vi "Save Data.vi"(8 "Sample ID":string, 9 "Channels":i32[](array[numeric]), 10 "Standard Input":T1, 11 "Input Data Arrays":T2) -> (3 "Output":string)   [LabVIEW 2017]
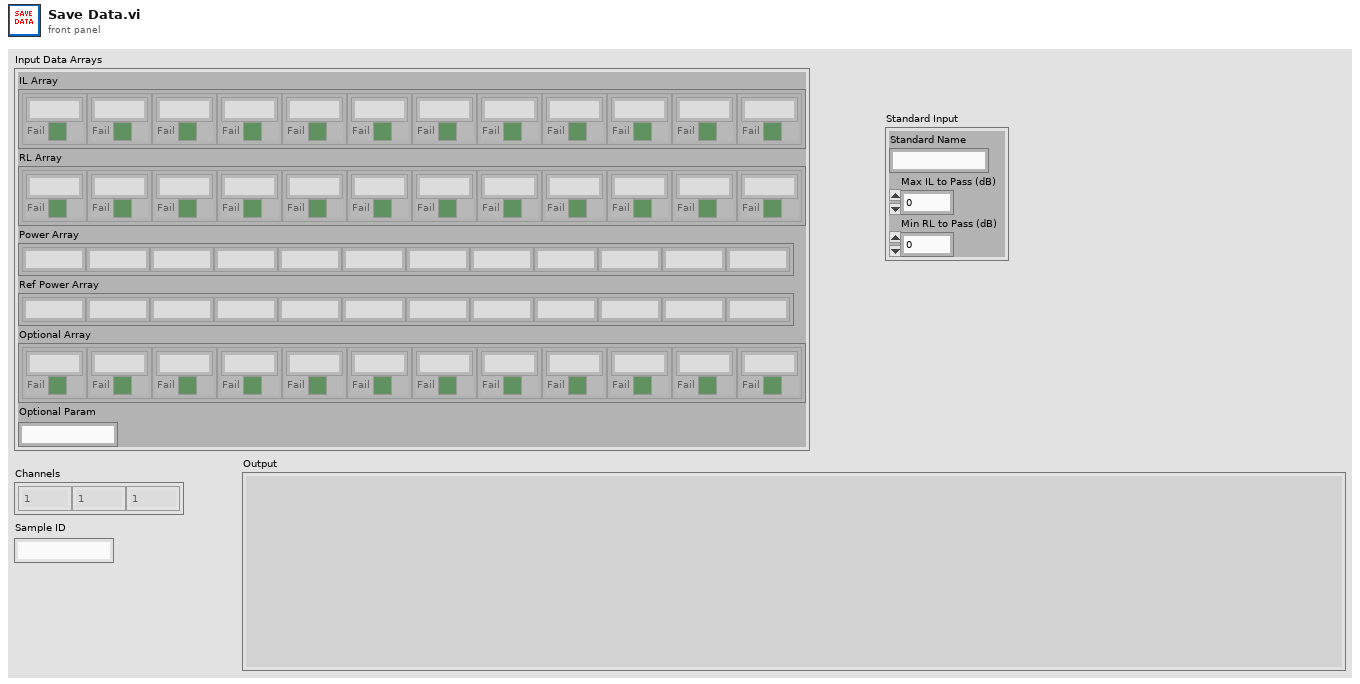
[diagram p1: front panel]
types:
  T1 = cluster{"Standard Name":string, "Max IL to Pass (dB)":dbl, "Min RL to Pass (dB)":dbl}
  T2 = cluster{"IL Array":cluster{"Data Output":string, "Fail":bool}[], "RL Array":cluster{"Data Output":string, "Fail":bool}[], "Power Array":string[], "Ref Power Array":string[], "Optional Array":cluster{"Data Output":string, "Fail":bool}[], "Optional Param":string}
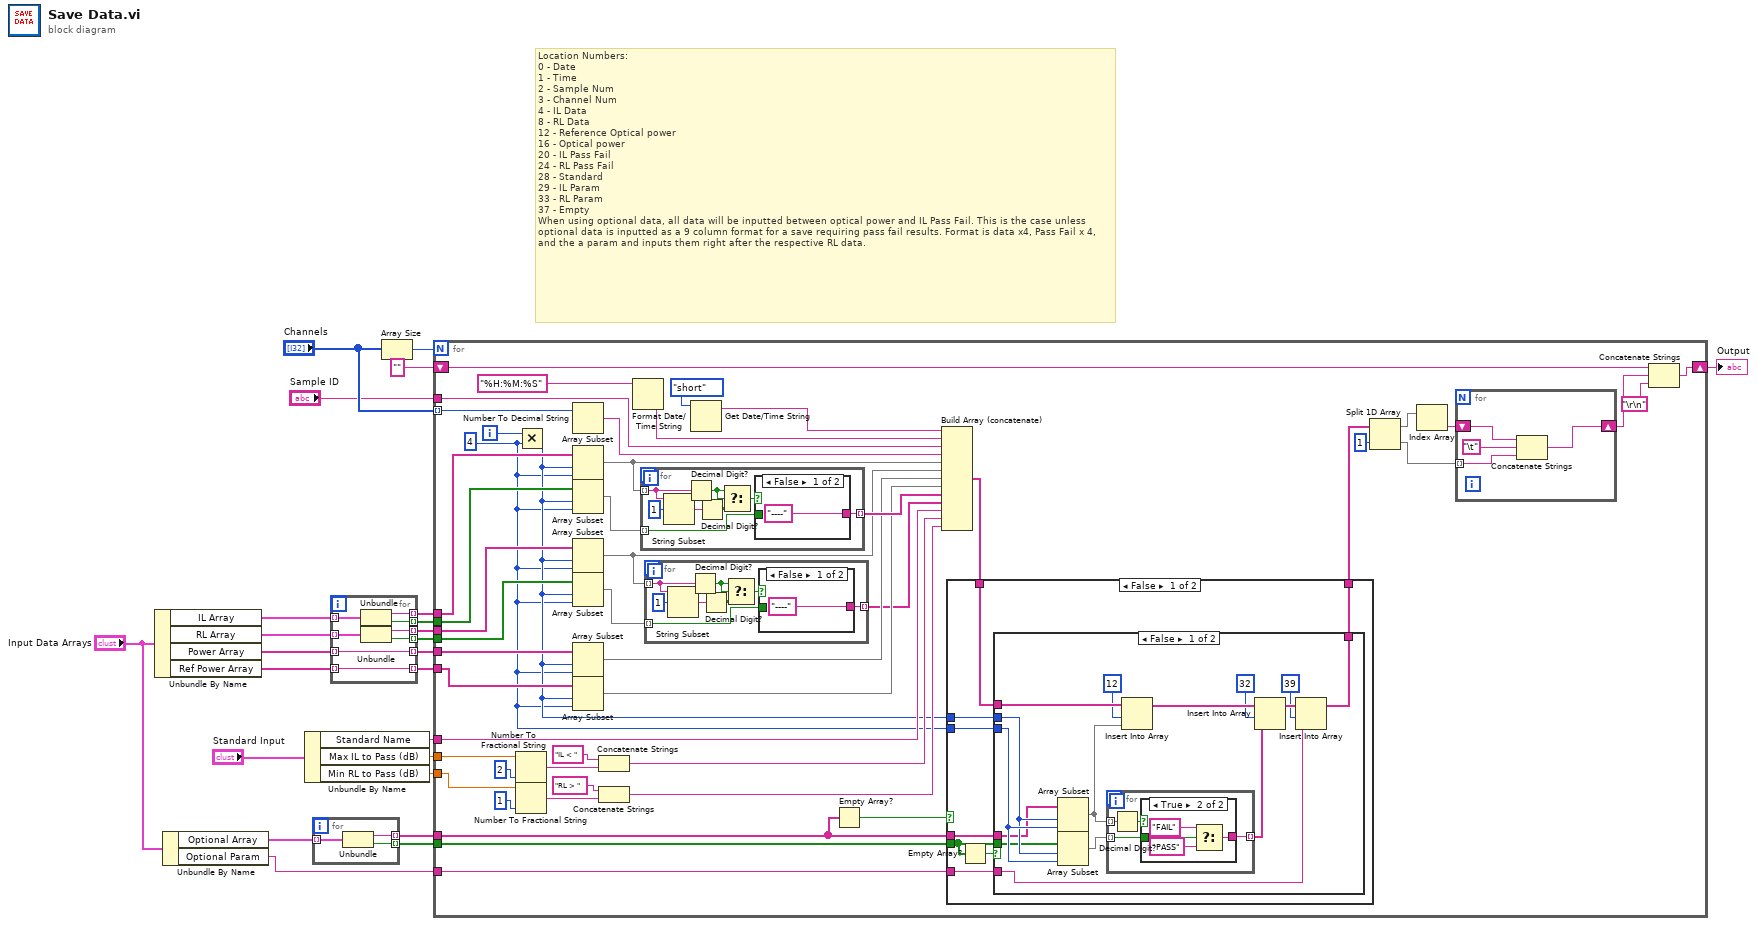
[diagram p0: block diagram]
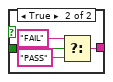
[diagram p2: hidden frame]
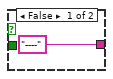
[diagram p3: hidden frame]
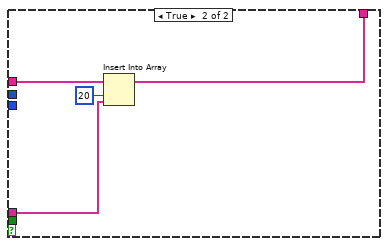
[diagram p4: hidden frame]
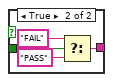
[diagram p6: hidden frame]
diagram:
  # "Location Numbers:\n0 - Date\n1 - Time\n2 - Sample Num\n3 - Channel Num\n4 - IL Data\n8 - RL Data\n12 - Reference Optical power\n16 - Optical power\n20 - IL Pass Fail\n24 - RL Pass Fail\n28 - Standard\n29 - IL Param\n33 - RL Param\n37 - Empty \nWhen using optional data, all data will be inputted between optical power and IL Pass Fail. This is the case unless optional data is inputted as a 9 column format for a save requiring pass fail results. Format is data x4, Pass Fail x 4, and the a param and inputs them right after the respective RL data."
  n1 = Unbundle By Name("Input Data Arrays") -> ("IL Array"=w19:cluster{"Data Output":string, "Fail":bool}[], "RL Array"=w18:cluster{"Data Output":string, "Fail":bool}[], "Power Array"=w16:string[], "Ref Power Array"=w17:string[])
  n2 = Unbundle By Name("Input Data Arrays") -> ("Optional Array"=w6:cluster{"Data Output":string, "Fail":bool}[], "Optional Param"=w5:string)
  n3 = Unbundle By Name("Standard Input") -> ("Standard Name"=w2:string, "Max IL to Pass (dB)"=w8:dbl, "Min RL to Pass (dB)"=w9:dbl)
  n4 = for {
    tunnel: w6 -> [w27] mode=indexing
    tunnel: [w26] -> w3 mode=indexing
    tunnel: [w25] -> w4 mode=indexing
    n5 = Unbundle(w27) -> ("Data Output"=w26:string, "Fail"=w25:bool)
  }
  n6 = for {
    tunnel: w19 -> [w35] mode=indexing
    tunnel: w18 -> [w34] mode=indexing
    tunnel: w17 -> [w32] mode=indexing
    tunnel: w16 -> [w33] mode=indexing
    tunnel: [w33] -> w11 mode=indexing
    tunnel: [w32] -> w10 mode=indexing
    tunnel: [w31] -> w15 mode=indexing
    tunnel: [w30] -> w14 mode=indexing
    tunnel: [w29] -> w13 mode=indexing
    tunnel: [w28] -> w12 mode=indexing
    n7 = Unbundle(w35) -> ("Data Output"=w31:string, "Fail"=w30:bool)
    n8 = Unbundle(w34) -> ("Data Output"=w29:string, "Fail"=w28:bool)
  }
  n9 = Array Size(array="Channels") -> (size(s)=w23:i32)
  n10 = for {
    N: w23 -> [_]
    tunnel: "Sample ID" -> [w81]
    tunnel: "Channels" -> [w80] mode=indexing
    shift-right: [w53] -> w24
    shift-left: "" -> [w79]
    tunnel: w15 -> [w76]
    tunnel: w14 -> [w75]
    tunnel: w13 -> [w72]
    tunnel: w12 -> [w71]
    tunnel: w11 -> [w44]
    tunnel: w10 -> [w43]
    tunnel: w9 -> [w61]
    tunnel: w8 -> [w69]
    tunnel: w5 -> [w47]
    tunnel: w4 -> [w48]
    tunnel: w3 -> [w49]
    tunnel: w2 -> [w51]
    i -> [w82]
    w39 = 4
    n11 = Number To Fractional String(number=w69, precision (6)=i16 2) -> (F-format string=w66:string)  [unwired: 2 in]
    n12 = Number To Fractional String(number=w61, precision (6)=i16 1) -> (F-format string=w64:string)  [unwired: 2 in]
    n13 = Multiply(x=w82, y=w39) -> (x*y=w40:i32)
    n14 = Number To Decimal String(number=w80) -> (decimal integer string=w83:string)  [unwired: 1 in]
    n15 = Array Subset(array=w76, index=w40, length=w39) -> (w73:string[])
    n16 = Array Subset(array=w75, index=w40, length=w39) -> (w74:bool[])
    n17 = Array Subset(array=w72, index=w40, length=w39) -> (w38:string[])
    n18 = Array Subset(array=w71, index=w40, length=w39) -> (w37:bool[])
    n19 = Array Subset(array=w44, index=w40, length=w39) -> (w42:string[])
    n20 = Array Subset(array=w43, index=w40, length=w39) -> (w41:string[])
    n21 = Concatenate Strings("IL < ", w66) -> (w63:string)
    n22 = Concatenate Strings("RL > ", w64) -> (w62:string)
    n23 = Format Date/Time String(time format string (%c)="%H:%M:%S") -> (date/time string=w77:string)  [unwired: 2 in]
    n24 = for {
      tunnel: w74 -> [w146] mode=indexing
      tunnel: [w145] -> w52 mode=indexing
      tunnel: w73 -> [w139] mode=indexing
      n25 = String Subset(string=w139, offset (0)=1) -> (substring=w143:string)  [unwired: 1 in]
      n26 = Decimal Digit?(1:w139) -> (0:w141:bool)
      n27 = Decimal Digit?(1:w143) -> (0:w144:bool)
      n28 = Select(t=w141, s=w141, f=w144) -> (s? t:f=w140:bool)
      n29 = case shown="False" w140 {
        tunnel: w146 -> [_ w149]
        tunnel: ["----" w148] -> w145
        frame False {
        }
        frame True {
          n30 = Select(t="FAIL", s=w149, f="PASS") -> (s? t:f=w148:string)
        }
      }
    }
    n31 = for {
      tunnel: w37 -> [w92] mode=indexing
      tunnel: [w91] -> w36 mode=indexing
      tunnel: w38 -> [w85] mode=indexing
      n32 = String Subset(string=w85, offset (0)=1) -> (substring=w89:string)  [unwired: 1 in]
      n33 = Decimal Digit?(1:w85) -> (0:w87:bool)
      n34 = Decimal Digit?(1:w89) -> (0:w90:bool)
      n35 = Select(t=w87, s=w87, f=w90) -> (s? t:f=w86:bool)
      n36 = case shown="False" w86 {
        tunnel: w92 -> [_ w95]
        tunnel: ["----" w94] -> w91
        frame False {
        }
        frame True {
          n37 = Select(t="FAIL", s=w95, f="PASS") -> (s? t:f=w94:string)
        }
      }
    }
    n38 = Get Date/Time String(date format (0)=enum16{"short", "long", "abbreviated"}."short") -> (date string=w60:string)  [unwired: 2 in, 1 out]
    n39 = Empty Array?(array=w49) -> (empty?=w50:bool)
    n40 = Build Array (concatenate)(w60, w77, w81, w83, w73, w38, w42, w41, w52, w36, w51, w63, w62) -> (w45:string[])
    n41 = case shown="False" w50 {
      tunnel: w49 -> [w104 _]
      tunnel: w48 -> [w103 _]
      tunnel: w47 -> [w102 _]
      tunnel: [w100 w134] -> w46
      tunnel: w45 -> [w101 w134]
      tunnel: w39 -> [w99 _]
      tunnel: w40 -> [w98 _]
      frame False {
        n42 = Empty Array?(array=w103) -> (empty?=w105:bool)
        n43 = case shown="False" w105 {
          tunnel: w104 -> [w117 w133]
          tunnel: w103 -> [w116 _]
          tunnel: w102 -> [w106 _]
          tunnel: w101 -> [w113 w132]
          tunnel: [w112 w130] -> w100
          tunnel: w99 -> [w120 _]
          tunnel: w98 -> [w119 _]
          frame False {
            n44 = Array Subset(array=w117, index=w119, length=w120) -> (w108:string[])
            n45 = Array Subset(array=w116, index=w119, length=w120) -> (w118:bool[])
            n46 = for {
              tunnel: w118 -> [w124] mode=indexing
              tunnel: [w123] -> w107 mode=indexing
              tunnel: w108 -> [w122] mode=indexing
              n47 = Decimal Digit?(1:w122) -> (0:w121:bool)
              n48 = case shown="True" w121 {
                tunnel: w124 -> [_ w127]
                tunnel: ["----" w126] -> w123
                frame False {
                }
                frame True {
                  n49 = Select(t="FAIL", s=w127, f="PASS") -> (s? t:f=w126:string)
                }
              }
            }
            n50 = Insert Into Array(array=w113, index=12 ("index (row)"), new element=w108) -> (w115:string[])
            n51 = Insert Into Array(array=w115, index=32 ("index (row)"), new element=w107) -> (w114:string[])
            n52 = Insert Into Array(array=w114, index=39 ("index (row)"), new element=w106) -> (w112:string[])
          }
          frame True {
            n53 = Insert Into Array(array=w132, index=20 ("index (row)"), new element=w133) -> (w130:string[])
          }
        }
      }
      frame True {
      }
    }
    n54 = Split 1D Array(array=w46, index=1) -> (first subarray=w56:string[], second subarray=w58:string[])
    n55 = Index Array(array=w56) -> (element=w57:string)  [unwired: 1 in]
    n56 = for {
      tunnel: w58 -> [w138] mode=indexing
      shift-right: [w137] -> w55
      shift-left: w57 -> [w136]
      n57 = Concatenate Strings(w136, "\t", w138) -> (w137:string)
    }
    n58 = Concatenate Strings(w79, w55, "\r\n") -> (w53:string)
  }
  "Output" <- w24
